vi "login.vi"() -> ()   [LabVIEW 2015]
uses:
  Control Button/login.ctl
  <vilib>/addons/database/NI_Database_API.lvlib
  Trail/Global 1-01.vi
  <vilib>/addons/database/_DB Variant To Data/Database Variant To Data.xnode
  <vilib>/addons/database/Connection.llb/DB Tools Open Connec (String).vi
panel:
  out "x >= y?":bool
  out "date/time string":string
  out "Boolean":bool
  in  "LOgin":T1
  in  "User Type":enum16{"Admin", "Operator", "Manufacture"}(ring)
  in  "Password":string
  in  "User name":string
  out "error out":errorcluster
  out "empty?":bool
  out "user":string
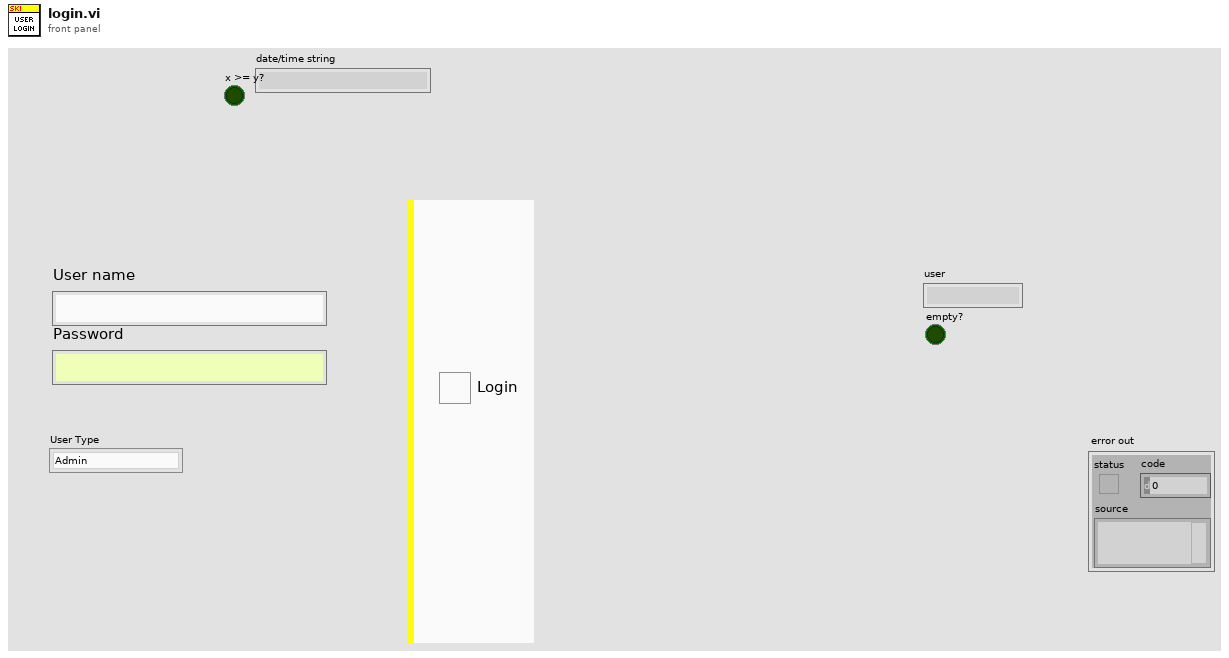
[diagram p1: front panel]
types:
  T1 = typedef "login.ctl" = bool
  T2 = typedef "NI_Database_API.lvlib/Conn ObjectReference.ctl" = refnum<k1>
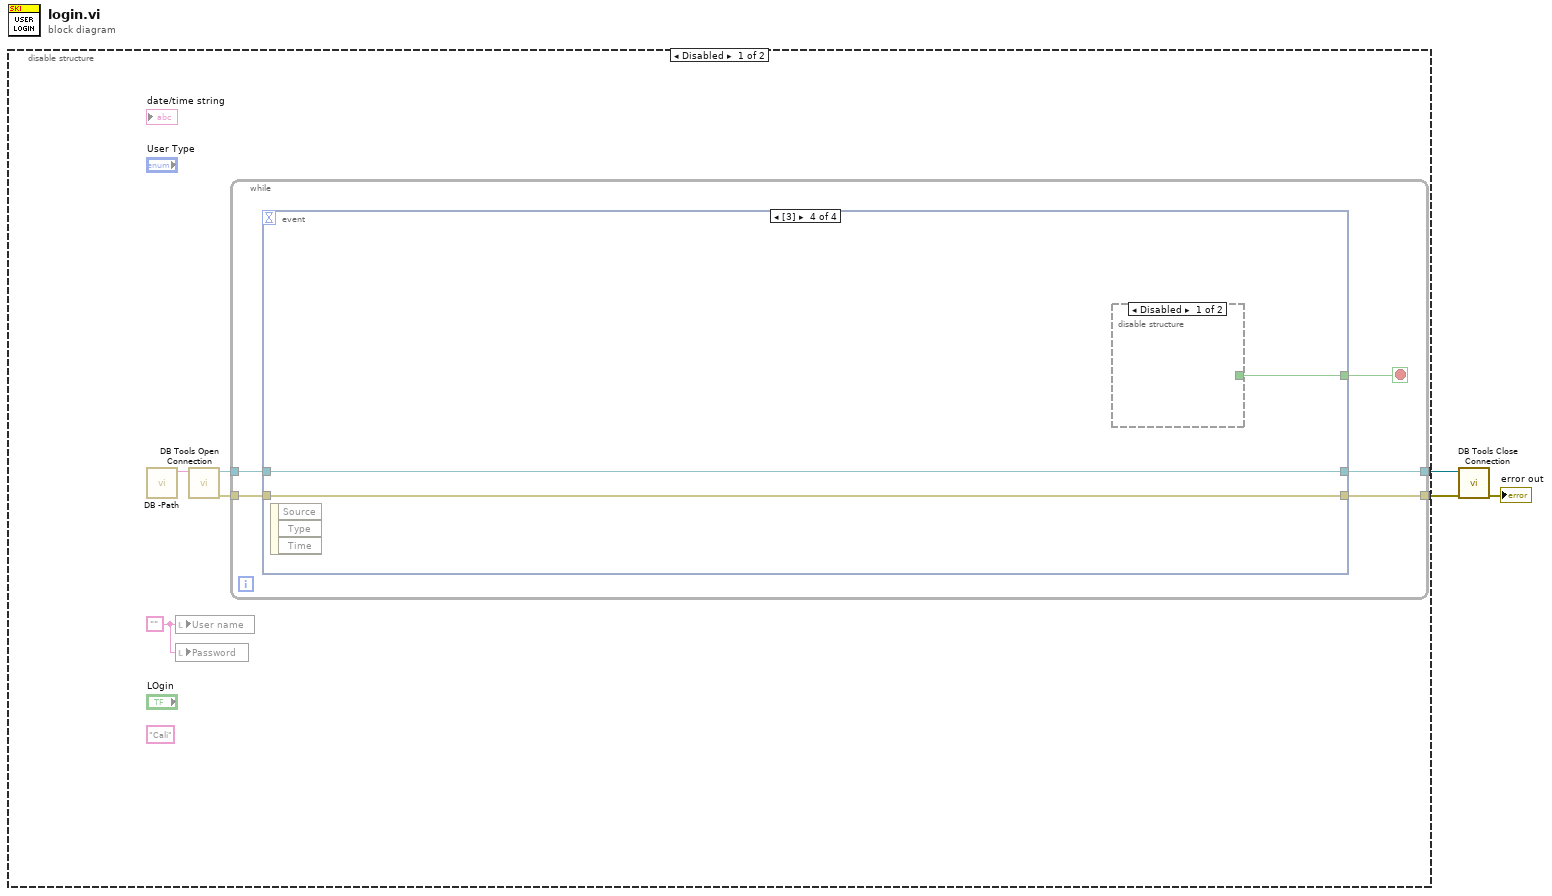
[diagram p0: block diagram]
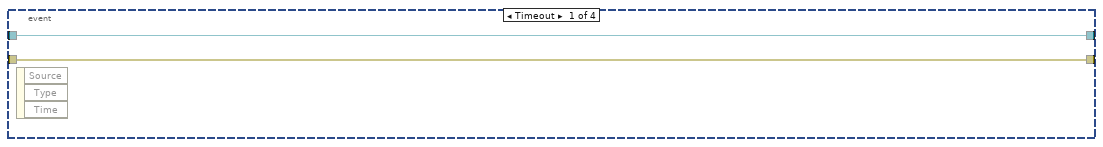
[diagram p2: hidden frame]
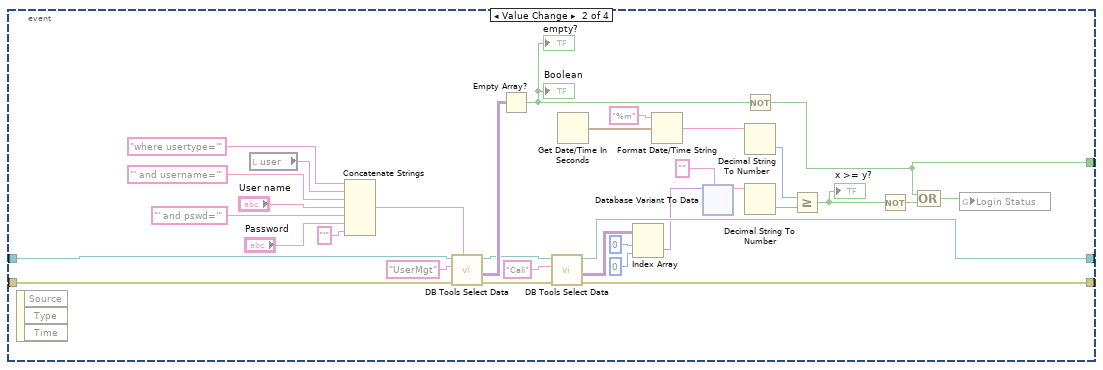
[diagram p3: hidden frame]
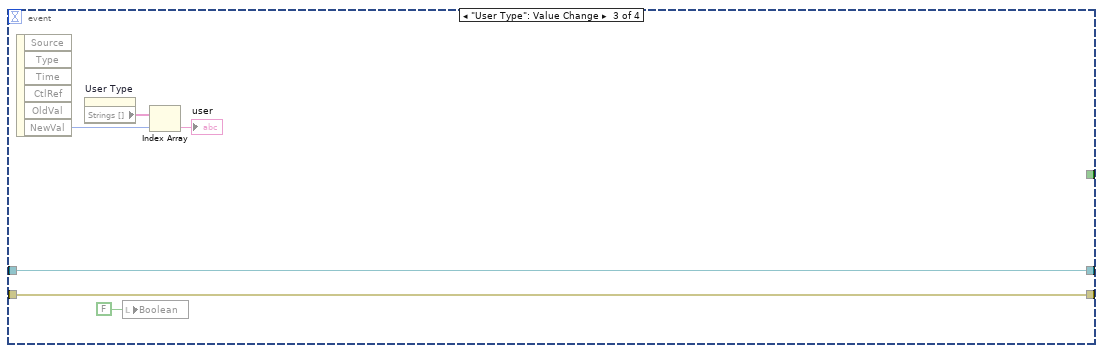
[diagram p4: hidden frame]
diagram:
  n1 = disable-structure shown="Disabled" {
    disable-tunnel: [w6 _] -> w3
    disable-tunnel: [w5 _] -> w2
    frame Disabled {
      w4 = ""
      (unwired) "Cali" ("table")
      n2 = call "DB -Path.vi"() -> ("String"=w9:string)  [unwired: 11 in]
      n3 = local write "User name"(w4) -> ()
      n4 = local write "Password"(w4) -> ()
      n5 = call-poly <vilib>:"DB Tools Open Connection.vi"("connection information"=w9) -> ("error out"=w7:errorcluster, "connection reference"=w8:T2)  [unwired: 7 in]
      n6 = while {
        tunnel: w8 -> [w13]
        tunnel: w7 -> [w12]
        tunnel: [w11] -> w6
        tunnel: [w10] -> w5
        stop <- w14 stop-if-true
        n7 = event shown="[3]" {
          selector: _ -> [_ _ _ _]
          dyn-events: _ -> [_ _ _ _]
          timeout: _ -> [_ _ _ _]
          tunnel: [_ w24 _ w90] -> w14
          tunnel: w13 -> [w16 w49 w83 w89]
          tunnel: w12 -> [w15 w48 w82 w88]
          tunnel: [w16 w33 w83 w89] -> w11
          tunnel: [w15 w32 w82 w88] -> w10
          event Timeout {
            n8 = event-data() -> ()  [unwired: 1 in, 3 out]
          }
          event Value Change {
            n9 = event-data() -> ()  [unwired: 1 in, 3 out]
            n10 = local read "user"() -> (w42:string)
            n11 = Concatenate Strings("where usertype='" ("condition"), w42, "' and username='" ("string"), "User name", "' and pswd='" ("string"), "Password", "'" ("string")) -> (w39:string)
            n12 = call <vilib>:"DB Tools Select Data.vi"("condition"=w39, "error in (no error)"=w48, "table"="UserMgt", "connection reference"=w49) -> ("error out"=w35:errorcluster, "data"=w38:variant[][], "connection reference out"=w36:T2)  [unwired: 2 in]
            n13 = Empty Array?(array=w38) -> (empty?=w37:bool)
            "empty?" <- w37
            "Boolean" <- w37
            n14 = call <vilib>:"DB Tools Select Data.vi"("error in (no error)"=w35, "table"="Cali", "connection reference"=w36) -> ("error out"=w32:errorcluster, "data"=w30:variant[][], "connection reference out"=w33:T2)  [unwired: 3 in]
            n15 = Get Date/Time In Seconds() -> (seconds since 1Jan1904=w26:timestamp)
            n16 = Index Array(array=w30, index (row)=0, index (col)=0 ("disabled index (col)")) -> (element=w29:variant)
            n17 = Format Date/Time String(time format string (%c)="%m", seconds (now)=w26) -> (date/time string=w21:string)  [unwired: 1 in]
            n18 = xnode "Database Variant To Data"("database variant"=w29, "type"="") -> ("data"=w23:string)  [unwired: 1 in, 1 out]
            n19 = Not(x=w37) -> (.not. x?=w24:bool)
            n20 = Decimal String To Number(string=w21) -> (number=w20:i32)  [unwired: 2 in, 1 out]
            n21 = Decimal String To Number(string=w23) -> (number=w22:i32)  [unwired: 2 in, 1 out]
            n22 = Greater Or Equal?(x=w20, y=w22) -> (x >= y?=w19:bool)
            "x >= y?" <- w19
            n23 = Not(x=w19) -> (.not. x?=w18:bool)
            n24 = Compound Arithmetic op=OR(w24, w18) -> (w17:bool)
            n25 = global write "Global 1-01.vi" "Login Status"(w17) -> ()
          }
          event "User Type": Value Change {
            n26 = event-data() -> ("NewVal"=w86:enum16{"Admin", "Operator", "Manufacture"})  [unwired: 1 in, 5 out]
            n27 = property on="User Type" class="Enum (strict)"() -> ("Strings []"=w87:string[])  [unwired: 2 in, 2 out]
            n28 = local write "Boolean"(FALSE ("Boolean")) -> ()
            n29 = Index Array(array=w87, index=w86) -> (element=→"user":string)
          }
          event #3 (no event record) {
            n30 = event-data() -> ()  [unwired: 1 in, 3 out]
            n31 = disable-structure shown="Disabled" {
              disable-tunnel: [w91 _] -> w90
              frame Disabled {
              }
              frame Enabled {
              }
            }
          }
        }
      }
    }
    frame Enabled {
    }
  }
  n32 = call <vilib>:"DB Tools Close Connection.vi"("error in (no error)"=w2, "connection reference"=w3) -> ("error out"=→"error out":errorcluster)  [unwired: 5 in]
